vi "串口事件.vi"() -> ()   [LabVIEW 2012]
panel:
  out "数字(0-1)":dbl
  in  "随机数":string
  in  "停止":bool
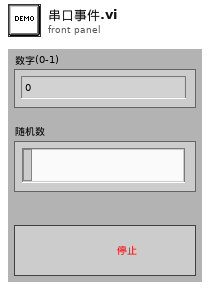
[diagram p1: front panel]
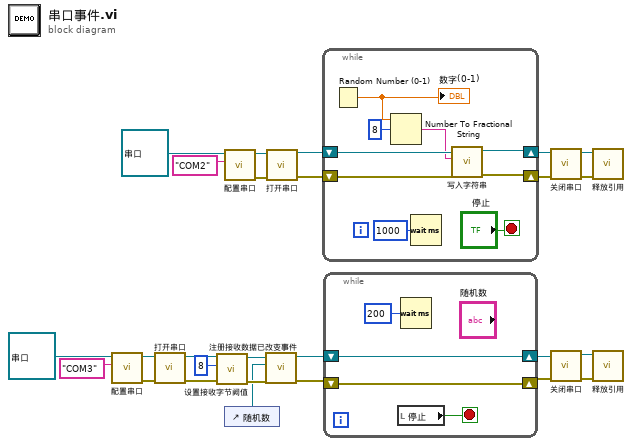
[diagram p0: block diagram]
diagram:
  n1 = call "配置串口.vi"("Port Name"="COM3", "COM 输入"=refnum<class "串口.lvclass"> refnum ("串口.lvclass")) -> ("error out"=w8:errorcluster, "COM 输出"=w9:refnum<class "串口.lvclass">)  [unwired: 8 in]
  n2 = call "打开串口.vi"("error in (no error)"=w8, "串口 输入"=w9) -> ("error out"=w11:errorcluster, "串口 输出"=w12:refnum<class "串口.lvclass">)  [unwired: 8 in]
  n3 = call "设置接收字节阙值.vi"("error in (no error)"=w11, "ReceivedBytesThreshold"=8, "串口 输入"=w12) -> ("error out"=w6:errorcluster, "串口 输出"=w7:refnum<class "串口.lvclass">)  [unwired: 7 in]
  n4 = call "配置串口.vi"("Port Name"="COM2", "COM 输入"=refnum<class "串口.lvclass"> refnum ("串口.lvclass")) -> ("error out"=w23:errorcluster, "COM 输出"=w24:refnum<class "串口.lvclass">)  [unwired: 8 in]
  n5 = control-ref of="随机数"() -> (w5:refnum<vi>)
  n6 = call "注册接收数据已改变事件.vi"("error in (no error)"=w6, "Ctl引用句柄"=w5, "串口 输入"=w7) -> ("error out"=w2:errorcluster, "串口 输出"=w4:refnum<class "串口.lvclass">)  [unwired: 7 in]
  n7 = call "打开串口.vi"("error in (no error)"=w23, "串口 输入"=w24) -> ("error out"=w21:errorcluster, "串口 输出"=w22:refnum<class "串口.lvclass">)  [unwired: 8 in]
  n8 = while {
    shift-right: [w31] -> w19
    shift-left: w21 -> [w32]
    shift-right: [w34] -> w20
    shift-left: w22 -> [w33]
    stop <- "停止" stop-if-true
    n9 = Random Number (0-1)() -> (number: 0 to 1=w29:dbl)
    "数字(0-1)" <- w29
    n10 = Number To Fractional String(number=w29, width (-)=i16 8 ("宽度(-)")) -> (F-format string=w28:string)  [unwired: 2 in]
    n11 = Wait (ms)(milliseconds to wait=u32 1000 ("等待时间（毫秒）")) -> ()  [unwired: 1 out]
    n12 = call "写入字符串.vi"("error in (no error)"=w32, "字符串"=w28, "串口 输入"=w33) -> ("error out"=w31:errorcluster, "串口 输出"=w34:refnum<class "串口.lvclass">)  [unwired: 7 in]
  }
  n13 = while {
    shift-right: [w39] -> w3
    shift-left: w4 -> [w39]
    shift-right: [w38] -> w1
    shift-left: w2 -> [w38]
    stop <- w37 stop-if-true
    n14 = local read "停止"() -> (w37:bool)
    n15 = Wait (ms)(milliseconds to wait=u32 200 ("等待时间（毫秒）")) -> ()  [unwired: 1 out]
  }
  n16 = call "关闭串口.vi"("error in (no error)"=w19, "串口 输入"=w20) -> ("error out"=w18:errorcluster, "串口 输出"=w17:refnum<class "串口.lvclass">)  [unwired: 8 in]
  n17 = call "关闭串口.vi"("error in (no error)"=w1, "串口 输入"=w3) -> ("error out"=w13:errorcluster, "串口 输出"=w14:refnum<class "串口.lvclass">)  [unwired: 8 in]
  n18 = call "释放引用.vi"("error in (no error)"=w18, "串口 输入"=w17) -> ()  [unwired: 8 in, 2 out]
  n19 = call "释放引用.vi"("error in (no error)"=w13, "串口 输入"=w14) -> ()  [unwired: 8 in, 2 out]
